vi "Teleop.vi"(10 "Match Info":T1={"Autonomous Elapsed Seconds"=0.0, "TeleOp Elapsed Seconds"=0.0, "Disabled Elapsed Seconds"=0.0, "Visited Autonomous"=FALSE, "Visited TeleOp"=FALSE, "Visited Disabled"=FALSE, "Autonomous Settings"={"Autonomous Style"=enum."Independent", "VI Refnum"=refnum}}, 11 "Call Context":T2) -> ()   [LabVIEW 2011]
doc: "This VI is called for each TeleOp packet received from the DS where the robot is not disabled. It is often used to read from the joysticks and update I/O or to update setpoints for timed control loops. It should complete and return within 20 milliseconds or it may miss DS packets."
uses:
  <vilib>/Rock Robotics/WPI/DriverStation/WPI_DriverStationDerivedRobotMode.ctl
  <vilib>/Rock Robotics/WPI/DriverStation/WPI_DriverStationMatch Info.ctl
  <vilib>/Rock Robotics/WPI/Relay/WPI_RelayValue.ctl
  <vilib>/Rock Robotics/WPI/DriverStation/DriverStationLCD/WPI_DriverStationLCDLCDLine.ctl
  GLOBALMain.vi
  GLOBALHarvester.vi
  GLOBALShooter.vi
  GLOBALBridge.vi
  GLOBALDriveTrain.vi
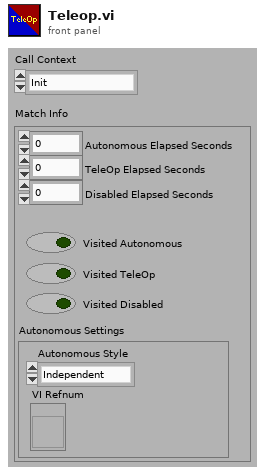
[diagram p1: front panel]
types:
  T1 = typedef "WPI_DriverStationMatch Info.ctl" = cluster{"Autonomous Elapsed Seconds":dbl, "TeleOp Elapsed Seconds":dbl, "Disabled Elapsed Seconds":dbl, "Visited Autonomous":bool, "Visited TeleOp":bool, "Visited Disabled":bool, "Autonomous Settings":cluster{"Autonomous Style":enum16{"Iterative", "Independent"}, "VI Refnum":refnum<vi>}}
  T2 = typedef "WPI_DriverStationDerivedRobotMode.ctl" = enum16{"Init", "Execute", "Stop"}
  T3 = typedef "WPI_RelayValue.ctl" = enum16{"Off", "On", "Forward", "Reverse"}
  T4 = typedef "WPI_RelayDevRef.ctl" = cluster{"DevStatus":errorcluster, "Relay Channel":T5, "Digital Module":T6, "Relay Direction":T7}
  T5 = typedef "FPGA_DIORelayChannel.ctl" = enum8{"Relay 1", "Relay 2", "Relay 3", "Relay 4", "Relay 5", "Relay 6", "Relay 7", "Relay 8", "Invalid"}
  T6 = typedef "FPGA_TypedefDigitalModule.ctl" = enum16{"Digital Module 1", "Digital Module 2"}
  T7 = typedef "WPI_RelayDirection.ctl" = enum16{"Both directions", "Forward only", "Reverse only"}
  T8 = cluster{"Driver Station Digital Input (1-8)[0]":bool, "Driver Station Digital Input (1-8)[1]":bool, "Driver Station Digital Input (1-8)[2]":bool, "Driver Station Digital Input (1-8)[3]":bool, "Driver Station Digital Input (1-8)[4]":bool, "Driver Station Digital Input (1-8)[5]":bool, "Driver Station Digital Input (1-8)[6]":bool, "Driver Station Digital Input (1-8)[7]":bool, "Driver Station Digital Input (1-8)[8]":bool}
  T9 = typedef "WPI_JoystickDevRef.ctl" = cluster{"Device":T10}
  T10 = typedef "WPI_JoystickDeviceEnum.ctl" = enum16{"USB 1", "USB 2", "USB 3", "USB 4", "Kinect 1", "Kinect 2"}
  T11 = typedef "WPI_JoystickButtonState.ctl" = cluster{"Button 1":bool, "Button 2":bool, "Button 3":bool, "Button 4":bool, "Button 5":bool, "Button 6":bool, "Button 7":bool, "Button 8":bool, "Button 9":bool, "Button 10":bool, "Button 11":bool, "Button 12":bool}
  T12 = typedef "WPI_EncoderDevRef.ctl" = cluster{"DevStatus":errorcluster, "EncoderIndex":T13, "CounterIndex":T14, "DistancePerCount":dbl, "Decoding Type":T15}
  T13 = typedef "FPGA_EncoderIdx.ctl" = enum8{"Enc 0", "Enc 1", "Enc 2", "Enc 3", "Invalid"}
  T14 = typedef "FPGA_CounterCtrSystemIndex.ctl" = enum8{"Ctr 0", "Ctr 1", "Ctr 2", "Ctr 3", "Ctr 4", "Ctr 5", "Ctr 6", "Ctr 7", "Invalid"}
  T15 = typedef "WPI_EncoderType.ctl" = enum16{"1x", "2x", "4x"}
  T16 = cluster{"axis 1 (x)":dbl, "axis 2 (y)":dbl, "axis 3 (throttle)":dbl, "axis 4":dbl, "axis 5":dbl, "axis 6":dbl}
  T17 = cluster{"Shifting":cluster{"Right Servo High":dbl, "Right Servo Low":dbl, "Left Servo High":dbl, "Left Servo Low":dbl}, "Breaking":cluster{"Coast Position":dbl, "Break Position":dbl}}
  T18 = typedef "WPI_DriverStationLCDLCDLine.ctl" = enum16{"Main - Line 1", "User - Line 2", "User - Line 3", "User - Line 4", "User - Line 5", "User - Line 6"}
  T19 = typedef "WPI_DigitalInputDevRef.ctl" = cluster{"DevStatus":errorcluster, "DIO Channel":T20, "Digital Module":T6}
  T20 = typedef "FPGA_DIOChannel.ctl" = enum8{"DIO 1", "DIO 2", "DIO 3", "DIO 4", "DIO 5", "DIO 6", "DIO 7", "DIO 8", "DIO 9", "DIO 10", "DIO 11", "DIO 12", "DIO 13", "DIO 14", "Invalid"}
  T21 = typedef "WPI_ServoDeviceRef.ctl" = cluster{"DeviceStatus":errorcluster, "Digital Module":T6, "PWM Channel":T22, "DeadBand":T23}
  T22 = typedef "FPGA_DIOPWMChannel.ctl" = enum8{"PWM 1", "PWM 2", "PWM 3", "PWM 4", "PWM 5", "PWM 6", "PWM 7", "PWM 8", "PWM 9", "PWM 10", "Invalid"}
  T23 = typedef "WPI_PWMDeadband.ctl" = cluster{"Name":string, "maxPositivePwm":i32, "minPositivePwm":i32, "centerPwm":i32, "maxNegativePwm":i32, "minNegativePwm":i32, "angularRange":u16}
  T24 = typedef "WPI_MotorControlDeviceRef.ctl" = cluster{"DeviceStatus":errorcluster, "Type":enum16{"PWM", "CAN"}, "PWM":cluster{"Digital Module":T6, "PWM Channel":T22, "DeadBand":T23}, "CAN":cluster{"Device Number":u8, "Control Mode":T25, "Semaphore":T26, "Max Vout":dbl}, "Invert":bool, "TransformRef":T27, "InvTransformRef":T27}
  T25 = typedef "WPI_CANJaguar_ControlMode.ctl" = enum8{"Percent VBus", "Current", "Speed", "Position", "Voltage"}
  T26 = typedef "Semaphore RefNum" = refnum<k1>
  T27 = typedef "WPI_PWMTransform_ConPane.ctl" = refnum<vi>
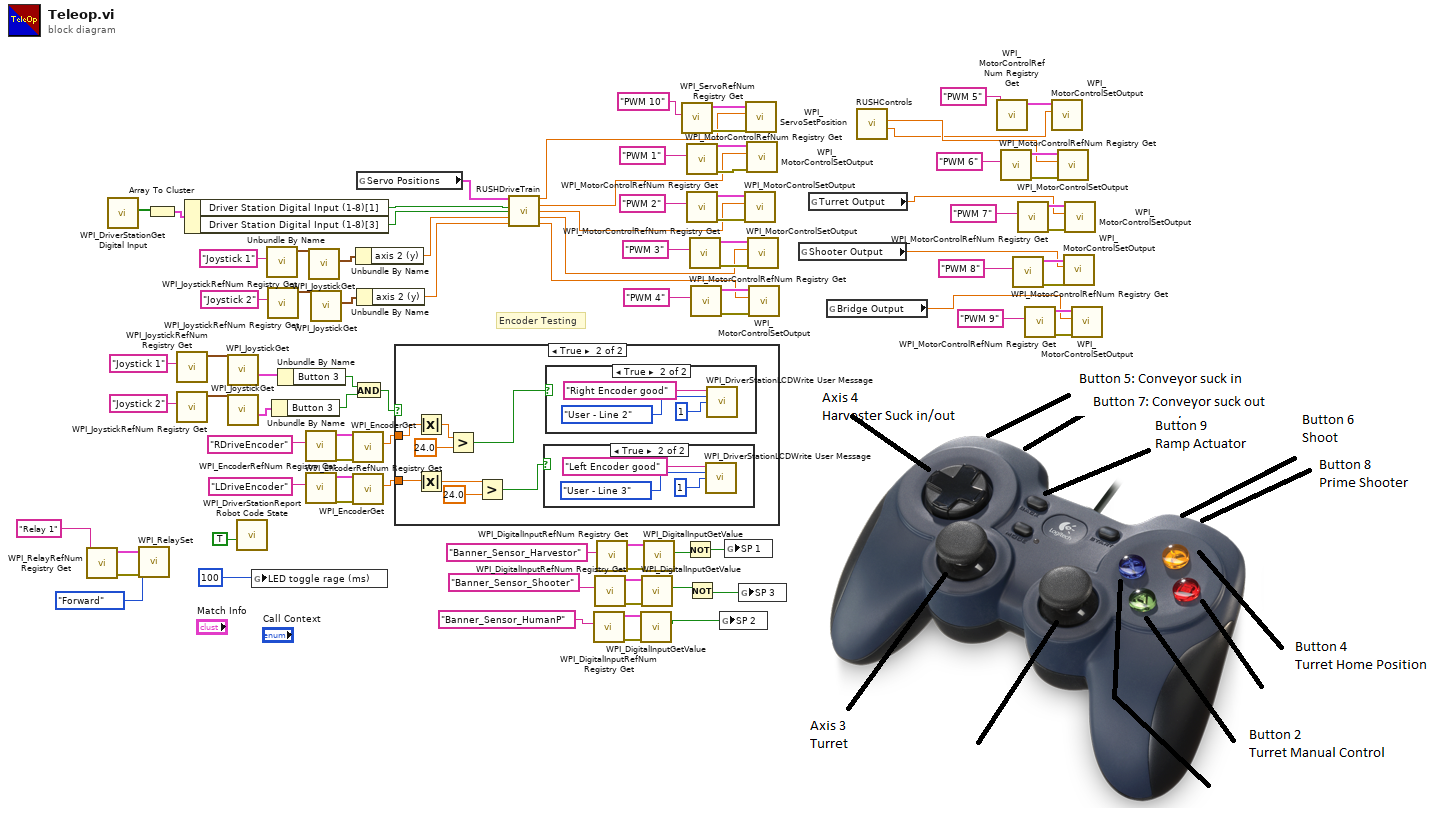
[diagram p0: block diagram]
diagram:
  # "Encoder Testing"
  n1 = call <vilib>:"WPI_RelayRefNum Registry Get.vi"("refnum name"="Relay 1") -> ("error out"=w78:errorcluster, "RelayDevRef"=w79:T4)  [unwired: 9 in]
  n2 = call <vilib>:"WPI_DriverStationGet Digital Input.vi"() -> ("Driver Station Digital Input (1-8)"=w32:bool[])  [unwired: 11 in]
  n3 = call <vilib>:"WPI_RelaySet.vi"("error in (no error)"=w78, "RelayValue"=WPI_RelayValue."Forward", "RelayDevRef"=w79) -> ()  [unwired: 7 in, 2 out]
  n4 = Array To Cluster(array=w32) -> (cluster=w31:T8)
  n5 = call <vilib>:"WPI_JoystickRefNum Registry Get.vi"("refnum name"="Joystick 1") -> ("JoystickDevRef"=w87:T9)  [unwired: 9 in, 1 out]
  n6 = call <vilib>:"WPI_JoystickRefNum Registry Get.vi"("refnum name"="Joystick 2") -> ("JoystickDevRef"=w86:T9)  [unwired: 9 in, 1 out]
  n7 = Unbundle By Name(w31) -> ("Driver Station Digital Input (1-8)[1]"=w30:bool, "Driver Station Digital Input (1-8)[3]"=w29:bool)
  n8 = call <vilib>:"WPI_JoystickGet.vi"("JoystickDevRef"=w87) -> ("Buttons"=w55:T11)  [unwired: 4 in, 2 out]
  n9 = call <vilib>:"WPI_JoystickGet.vi"("JoystickDevRef"=w86) -> ("Buttons"=w56:T11)  [unwired: 4 in, 2 out]
  n10 = call <vilib>:"WPI_DriverStationReport Robot Code State.vi"("TeleOp"=TRUE ("Autonomous")) -> ()  [unwired: 10 in, 1 out]
  n11 = global write "GLOBALMain.vi" "LED toggle rage (ms)"(u32 100 ("LED ms toggle rate")) -> ()
  n12 = call <vilib>:"WPI_JoystickRefNum Registry Get.vi"("refnum name"="Joystick 1") -> ("JoystickDevRef"=w27:T9)  [unwired: 9 in, 1 out]
  n13 = call <vilib>:"WPI_JoystickRefNum Registry Get.vi"("refnum name"="Joystick 2") -> ("JoystickDevRef"=w22:T9)  [unwired: 9 in, 1 out]
  n14 = Unbundle By Name(w56) -> ("Button 3"=w53:bool)
  n15 = Unbundle By Name(w55) -> ("Button 3"=w54:bool)
  n16 = call <vilib>:"WPI_EncoderRefNum Registry Get.vi"("refnum name"="RDriveEncoder") -> ("error out"=w49:errorcluster, "EncoderDevRef"=w50:T12)  [unwired: 9 in]
  n17 = call <vilib>:"WPI_EncoderRefNum Registry Get.vi"("refnum name"="LDriveEncoder") -> ("error out"=w48:errorcluster, "EncoderDevRef"=w47:T12)  [unwired: 9 in]
  n18 = call <vilib>:"WPI_JoystickGet.vi"("JoystickDevRef"=w27) -> ("Axes"=w28:T16)  [unwired: 4 in, 2 out]
  n19 = call <vilib>:"WPI_JoystickGet.vi"("JoystickDevRef"=w22) -> ("Axes"=w23:T16)  [unwired: 4 in, 2 out]
  n20 = call <vilib>:"WPI_EncoderGet.vi"("error in (no error)"=w49, "EncoderDevRef"=w50) -> ("Distance"=w45:dbl)  [unwired: 4 in, 5 out]
  n21 = call <vilib>:"WPI_EncoderGet.vi"("error in (no error)"=w48, "EncoderDevRef"=w47) -> ("Distance"=w44:dbl)  [unwired: 4 in, 5 out]
  n22 = And(x=w54, y=w53) -> (x .and. y?=w52:bool)
  n23 = Unbundle By Name(w28) -> ("axis 2 (y)"=w25:dbl)
  n24 = global read "GLOBALDriveTrain.vi" "Servo Positions"() -> (w33:T17)
  n25 = Unbundle By Name(w23) -> ("axis 2 (y)"=w21:dbl)
  n26 = case shown="True" w52 {
    tunnel: w45 -> [_ w92]
    tunnel: w44 -> [_ w91]
    frame False {
    }
    frame True {
      n27 = Absolute Value(x=w92) -> (abs(x)=w93:dbl)
      n28 = Absolute Value(x=w91) -> (abs(x)=w90:dbl)
      n29 = Greater?(x=w93, y=24.0) -> (0:w96:bool)
      n30 = Greater?(x=w90, y=24.0) -> (0:w94:bool)
      n31 = case shown="True" w94 {
        frame False {
        }
        frame True {
          n32 = call <vilib>:"WPI_DriverStationLCDWrite User Message.vi"("line text"="Left Encoder good", "line"=WPI_DriverStationLCDLCDLine."User - Line 3", "starting column"=i8 1) -> ()  [unwired: 2 in, 11 out]
        }
      }
      n33 = case shown="True" w96 {
        frame False {
        }
        frame True {
          n34 = call <vilib>:"WPI_DriverStationLCDWrite User Message.vi"("line text"="Right Encoder good", "line"=WPI_DriverStationLCDLCDLine."User - Line 2", "starting column"=i8 1) -> ()  [unwired: 2 in, 11 out]
        }
      }
    }
  }
  n35 = call "RUSHDriveTrain.vi"("Servo Positions"=w33, "Low Gear + Brake"=w30, "Low Gear"=w29, "LeftJoystick"=w25, "RightJoystick"=w21) -> ("Braking Servo"=w6:dbl, "Left Drive"=w5:dbl, "Right Drive"=w4:dbl, "Left Servo"=w3:dbl, "Right Servo"=w2:dbl)  [unwired: 6 in]
  n36 = call <vilib>:"WPI_DigitalInputRefNum Registry Get.vi"("refnum name"="Banner_Sensor_HumanP") -> ("error out"=w69:errorcluster, "DigitalInputDevRef"=w68:T19)  [unwired: 9 in]
  n37 = call <vilib>:"WPI_DigitalInputRefNum Registry Get.vi"("refnum name"="Banner_Sensor_Shooter") -> ("error out"=w70:errorcluster, "DigitalInputDevRef"=w71:T19)  [unwired: 9 in]
  n38 = call <vilib>:"WPI_DigitalInputRefNum Registry Get.vi"("refnum name"="Banner_Sensor_Harvestor") -> ("error out"=w73:errorcluster, "DigitalInputDevRef"=w72:T19)  [unwired: 9 in]
  n39 = call <vilib>:"WPI_DigitalInputGetValue.vi"("error in (no error)"=w69, "DigitalInputDevRef"=w68) -> ("Value"=w43:bool)  [unwired: 7 in, 2 out]
  n40 = call <vilib>:"WPI_DigitalInputGetValue.vi"("error in (no error)"=w70, "DigitalInputDevRef"=w71) -> ("Value"=w64:bool)  [unwired: 7 in, 2 out]
  n41 = call <vilib>:"WPI_DigitalInputGetValue.vi"("error in (no error)"=w73, "DigitalInputDevRef"=w72) -> ("Value"=w63:bool)  [unwired: 7 in, 2 out]
  n42 = call <vilib>:"WPI_ServoRefNum Registry Get.vi"("refnum name"="PWM 10") -> ("error out"=w14:errorcluster, "ServoDeviceRef"=w20:T21)  [unwired: 9 in]
  n43 = Not(x=w63) -> (.not. x?=w41:bool)
  n44 = call <vilib>:"WPI_MotorControlRefNum Registry Get.vi"("refnum name"="PWM 1") -> ("error out"=w16:errorcluster, "MotorControlDevRef"=w15:T24)  [unwired: 9 in]
  n45 = call <vilib>:"WPI_MotorControlRefNum Registry Get.vi"("refnum name"="PWM 2") -> ("error out"=w13:errorcluster, "MotorControlDevRef"=w17:T24)  [unwired: 9 in]
  n46 = Not(x=w64) -> (.not. x?=w42:bool)
  n47 = call <vilib>:"WPI_MotorControlRefNum Registry Get.vi"("refnum name"="PWM 3") -> ("error out"=w12:errorcluster, "MotorControlDevRef"=w8:T24)  [unwired: 9 in]
  n48 = call <vilib>:"WPI_MotorControlRefNum Registry Get.vi"("refnum name"="PWM 4") -> ("error out"=w9:errorcluster, "MotorControlDevRef"=w7:T24)  [unwired: 9 in]
  n49 = global write "GLOBALHarvester.vi" "SP 2"(w43) -> ()
  n50 = global write "GLOBALHarvester.vi" "SP 1"(w41) -> ()
  n51 = global write "GLOBALHarvester.vi" "SP 3"(w42) -> ()
  n52 = call <vilib>:"WPI_MotorControlSetOutput.vi"("error in (no error)"=w13, "Output"=w4, "MotorControlDevRef"=w17) -> ()  [unwired: 7 in, 2 out]
  n53 = call <vilib>:"WPI_ServoSetPosition.vi"("error in (no error)"=w14, "Position"=w6, "ServoDeviceRef"=w20) -> ()  [unwired: 7 in, 2 out]
  n54 = call <vilib>:"WPI_MotorControlSetOutput.vi"("error in (no error)"=w16, "Output"=w5, "MotorControlDevRef"=w15) -> ()  [unwired: 7 in, 2 out]
  n55 = call <vilib>:"WPI_MotorControlSetOutput.vi"("error in (no error)"=w12, "Output"=w3, "MotorControlDevRef"=w8) -> ()  [unwired: 7 in, 2 out]
  n56 = call <vilib>:"WPI_MotorControlSetOutput.vi"("error in (no error)"=w9, "Output"=w2, "MotorControlDevRef"=w7) -> ()  [unwired: 7 in, 2 out]
  n57 = global read "GLOBALShooter.vi" "Shooter Output"() -> (w38:dbl)
  n58 = global read "GLOBALShooter.vi" "Turret Output"() -> (w36:dbl)
  n59 = global read "GLOBALBridge.vi" "Bridge Output"() -> (w37:dbl)
  n60 = call "RUSHControls.vi"() -> ("Harvester"=w39:dbl, "Conveyor"=w40:dbl)  [unwired: 10 in]
  n61 = call <vilib>:"WPI_MotorControlRefNum Registry Get.vi"("refnum name"="PWM 5") -> ("MotorControlDevRef"=w74:T24)  [unwired: 9 in, 1 out]
  n62 = call <vilib>:"WPI_MotorControlRefNum Registry Get.vi"("refnum name"="PWM 6") -> ("error out"=w57:errorcluster, "MotorControlDevRef"=w58:T24)  [unwired: 9 in]
  n63 = call <vilib>:"WPI_MotorControlRefNum Registry Get.vi"("refnum name"="PWM 8") -> ("error out"=w61:errorcluster, "MotorControlDevRef"=w62:T24)  [unwired: 9 in]
  n64 = call <vilib>:"WPI_MotorControlRefNum Registry Get.vi"("refnum name"="PWM 7") -> ("error out"=w35:errorcluster, "MotorControlDevRef"=w80:T24)  [unwired: 9 in]
  n65 = call <vilib>:"WPI_MotorControlRefNum Registry Get.vi"("refnum name"="PWM 9") -> ("error out"=w83:errorcluster, "MotorControlDevRef"=w82:T24)  [unwired: 9 in]
  n66 = call <vilib>:"WPI_MotorControlSetOutput.vi"("Output"=w39, "MotorControlDevRef"=w74) -> ()  [unwired: 8 in, 2 out]
  n67 = call <vilib>:"WPI_MotorControlSetOutput.vi"("error in (no error)"=w57, "Output"=w40, "MotorControlDevRef"=w58) -> ()  [unwired: 7 in, 2 out]
  n68 = call <vilib>:"WPI_MotorControlSetOutput.vi"("error in (no error)"=w61, "Output"=w38, "MotorControlDevRef"=w62) -> ()  [unwired: 7 in, 2 out]
  n69 = call <vilib>:"WPI_MotorControlSetOutput.vi"("error in (no error)"=w35, "Output"=w36, "MotorControlDevRef"=w80) -> ()  [unwired: 7 in, 2 out]
  n70 = call <vilib>:"WPI_MotorControlSetOutput.vi"("error in (no error)"=w83, "Output"=w37, "MotorControlDevRef"=w82) -> ()  [unwired: 7 in, 2 out]
